vi "daemon.vi"(10 "queue":refnum<queue>, 11 "timer":refnum<queue>) -> ()   [LabVIEW 2017, in "rytimer.lvclass"]
uses:
  rytimer.lvclass
  enqueue.ctl
  state.ctl
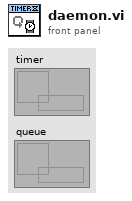
[diagram p1: front panel]
types:
  T1 = typedef "rytimer.lvclass/enqueue.ctl" = enum8{"back", "front", "back_if_absent", "front_if_absent"}
  T2 = cluster{"interval":u32, "message":string, "option":T1, "last":u32, "autoreset":bool, "run":bool}
  T3 = typedef "rytimer.lvclass/state.ctl" = enum8{"stop", "start", "mode", "interval", "message"}
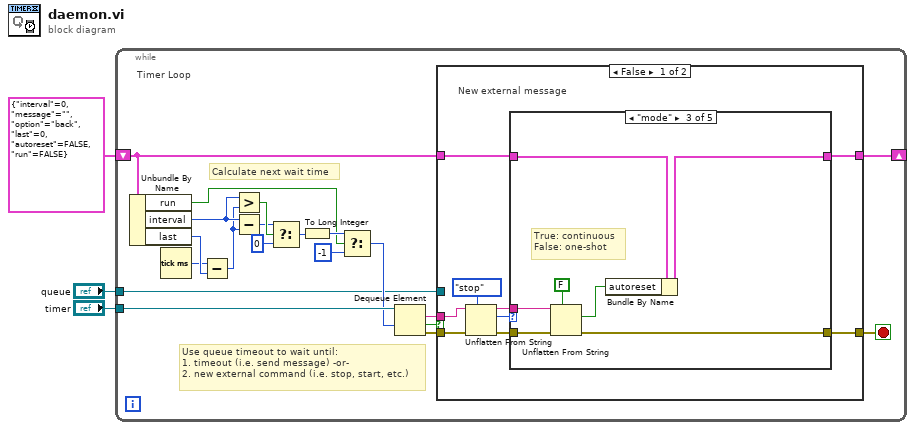
[diagram p0: block diagram]
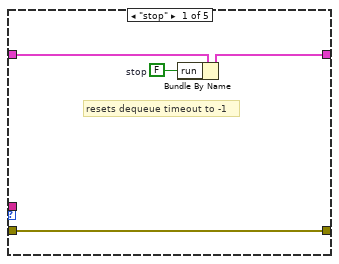
[diagram p2: hidden frame]
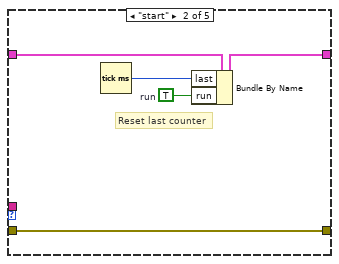
[diagram p3: hidden frame]
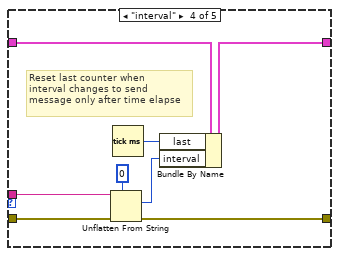
[diagram p4: hidden frame]
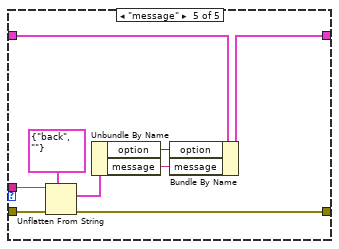
[diagram p5: hidden frame]
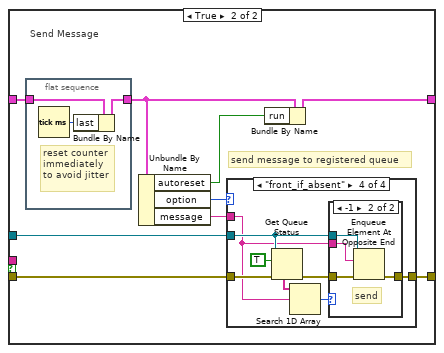
[diagram p6: hidden frame]
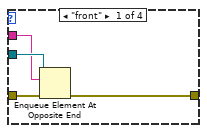
[diagram p7: hidden frame]
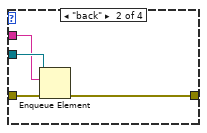
[diagram p8: hidden frame]
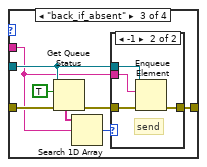
[diagram p9: hidden frame]
diagram:
  n1 = while {
    tunnel: "timer" -> [w23]
    shift-right: [w7] -> _
    shift-left: T2 {"interval"=0, "message"="", "option"=enum."back", "last"=0, "autoreset"=FALSE, "run"=FALSE} ("data") -> [w6]
    tunnel: "queue" -> [w4]
    stop <- w19 stop-if-true
    # "Use queue timeout to wait until:\n1. timeout (i.e. send message) -or-\n2. new external command (i.e. stop, start, etc.)"
    # "Calculate next wait time"
    # "Timer Loop"
    n2 = Unbundle By Name(w6) -> ("run"=w5:bool, "interval"=w14:u32, "last"=w15:u32)
    n3 = Tick Count (ms)() -> (millisecond timer value=w9:u32)
    n4 = Subtract(x=w9, y=w15) -> (x-y=w8:u32)
    n5 = Greater?(x=w14, y=w8) -> (0:w13:bool)
    n6 = Subtract(x=w14, y=w8) -> (x-y=w12:u32)
    n7 = Select(t=w12, s=w13, f=u32 0) -> (s? t:f=w10:u32)
    n8 = To Long Integer(number=w10) -> (32bit integer=w16:i32)
    n9 = Select(t=w16, s=w5, f=-1) -> (s? t:f=w17:i32)
    n10 = Dequeue Element(queue=w23, timeout in ms (-1)=w17) -> (element=w21:string, timed out?=w22:bool, error out=w20:errorcluster)  [unwired: 1 in, 1 out]
    n11 = case shown="False" w22 {
      tunnel: w21 -> [w30 _]
      tunnel: w20 -> [w31 w71]
      tunnel: [w24 w68] -> w7
      tunnel: w6 -> [w25 w74]
      tunnel: [w29 w70] -> w19
      tunnel: w4 -> [_ w66]
      frame False {
        # "New external message"
        n12 = Unflatten From String(type=state."stop" ("state"), binary string=w30, error in (no error)=w31) -> (rest of the binary string=w26:string, value=w27:T3, error out=w28:errorcluster)  [unwired: 2 in]
        n13 = case shown="\"mode\"" w27 {
          tunnel: [w36 w38 w44 w55 w61] -> w29
          tunnel: w28 -> [w36 w38 w48 w56 w65]
          tunnel: w26 -> [_ _ w47 w52 w64]
          tunnel: [w34 w40 w45 w54 w62] -> w24
          tunnel: w25 -> [w35 w41 w46 w53 w63]
          frame "stop" {
            w33 = FALSE  # stop
            # "resets dequeue timeout to -1"
            n14 = Bundle By Name(cluster=w35, "run"=w33) -> (w34:T2)
          }
          frame "start" {
            w37 = TRUE  # run
            # "Reset last counter"
            n15 = Tick Count (ms)() -> (millisecond timer value=w39:u32)
            n16 = Bundle By Name(cluster=w41, "last"=w39, "run"=w37) -> (w40:T2)
          }
          frame "mode" {
            # "True: continuous\nFalse: one-shot"
            n17 = Unflatten From String(type=FALSE, binary string=w47, error in (no error)=w48) -> (value=w43:bool, error out=w44:errorcluster)  [unwired: 2 in, 1 out]
            n18 = Bundle By Name(cluster=w46, "autoreset"=w43) -> (w45:T2)
          }
          frame "interval" {
            # "Reset last counter when\ninterval changes to send\nmessage only after time elapse"
            n19 = Unflatten From String(type=u32 0 ("interval"), binary string=w52, error in (no error)=w56) -> (value=w51:u32, error out=w55:errorcluster)  [unwired: 2 in, 1 out]
            n20 = Tick Count (ms)() -> (millisecond timer value=w50:u32)
            n21 = Bundle By Name(cluster=w53, "last"=w50, "interval"=w51) -> (w54:T2)
          }
          frame "message" {
            n22 = Unflatten From String(type=cluster{"option":T1, "message":string} {"option"=enum."back", "message"=""} ("output cluster"), binary string=w64, error in (no error)=w65) -> (value=w59:cluster{"option":T1, "message":string}, error out=w61:errorcluster)  [unwired: 2 in, 1 out]
            n23 = Unbundle By Name(w59) -> ("option"=w58:T1, "message"=w57:string)
            n24 = Bundle By Name(cluster=w63, "option"=w58, "message"=w57) -> (w62:T2)
          }
        }
      }
      frame True {
        # "send message to registered queue"
        # "Send Message"
        n25 = flat-sequence {
          tunnel: w74 -> [w77]
          tunnel: [w76] -> w69
          frame #0 {
            # "reset counter\nimmediately\nto avoid jitter"
            n26 = Tick Count (ms)() -> (millisecond timer value=w75:u32)
            n27 = Bundle By Name(cluster=w77, "last"=w75) -> (w76:T2)
          }
        }
        n28 = Unbundle By Name(w69) -> ("autoreset"=w67:bool, "option"=w72:T1, "message"=w73:string)
        n29 = case shown="\"front_if_absent\"" w72 {
          tunnel: w71 -> [w81 w85 w90 w103]
          tunnel: w66 -> [w80 w84 w89 w102]
          tunnel: w73 -> [w79 w83 w88 w101]
          tunnel: [w78 w82 w93 w106] -> w70
          frame "front" {
            n30 = Enqueue Element At Opposite End(queue=w80, element=w79, error in (no error)=w81) -> (error out=w78:errorcluster)  [unwired: 1 in, 2 out]
          }
          frame "back" {
            n31 = Enqueue Element(queue=w84, element=w83, error in (no error)=w85) -> (error out=w82:errorcluster)  [unwired: 1 in, 2 out]
          }
          frame "back_if_absent" {
            n32 = Get Queue Status(queue=w89, return elements? (F)=TRUE, error in (no error)=w90) -> (error out=w86:errorcluster, elements=w91:string[])  [unwired: 6 out]
            n33 = Search 1D Array(1D array=w91, element=w88) -> (index of element=w87:i32)  [unwired: 1 in]
            n34 = case shown="-1" w87 {
              tunnel: [w94 w98] -> w93
              tunnel: w89 -> [_ w97]
              tunnel: w88 -> [_ w96]
              tunnel: w86 -> [w94 w95]
              frame Default {
                # "msg\nexists,\ndrop"
              }
              frame -1 {
                # "send"
                n35 = Enqueue Element(queue=w97, element=w96, error in (no error)=w95) -> (error out=w98:errorcluster)  [unwired: 1 in, 2 out]
              }
            }
          }
          frame "front_if_absent" {
            n36 = Get Queue Status(queue=w102, return elements? (F)=TRUE, error in (no error)=w103) -> (error out=w99:errorcluster, elements=w104:string[])  [unwired: 6 out]
            n37 = Search 1D Array(1D array=w104, element=w101) -> (index of element=w100:i32)  [unwired: 1 in]
            n38 = case shown="-1" w100 {
              tunnel: [w107 w111] -> w106
              tunnel: w102 -> [_ w110]
              tunnel: w101 -> [_ w109]
              tunnel: w99 -> [w107 w108]
              frame Default {
                # "msg\nexists,\ndrop"
              }
              frame -1 {
                # "send"
                n39 = Enqueue Element At Opposite End(queue=w110, element=w109, error in (no error)=w108) -> (error out=w111:errorcluster)  [unwired: 1 in, 2 out]
              }
            }
          }
        }
        n40 = Bundle By Name(cluster=w69, "run"=w67) -> (w68:T2)
      }
    }
  }
